vi "SPC_set_adjust_parameters.vi"(6 "SPC Adjust Parameters":T1={"vrt1"=64, "vrt2"=128, "vrt3"=192, "dith_g"=128, "gain_1"=1.0, "gain_2"=1.0, "gain_4"=1.0, "gain_8"=1.0, "tac_r0"=1.0, "tac_r1"=1.0, "tac_r2"=1.0, "tac_r4"=1.0, "tac_r8"=1.0, "sync_div"=0} {"sync_div" min=0 max=2; "tac_r8" format="%.2f"; "tac_r4" format="%.2f"; "tac_r2" format="%.2f"; "tac_r1" format="%.2f"; "tac_r0" format="%.2f"; "gain_8" format="%.2f"; "gain_4" format="%.2f"; "gain_2" format="%.2f"; "gain_1" format="%.2f"}, 8 "Error In":errorcluster, 10 "Module No":i16 min=0 max=7 step=1, 11 "DLL Path":path) -> (0 "Error Out":errorcluster, 2 "Module No":i16 min=0 max=7 step=1, 3 "DLL Path":path, 4 "actualSPC Adjust Parameters":T1={"vrt1"=64, "vrt2"=128, "vrt3"=192, "dith_g"=128, "gain_1"=1.0, "gain_2"=1.0, "gain_4"=1.0, "gain_8"=1.0, "tac_r0"=1.0, "tac_r1"=1.0, "tac_r2"=1.0, "tac_r4"=1.0, "tac_r8"=1.0, "sync_div"=0} {"sync_div" min=0 max=2; "tac_r8" format="%.2f"; "tac_r4" format="%.2f"; "tac_r2" format="%.2f"; "tac_r1" format="%.2f"; "tac_r0" format="%.2f"; "gain_8" format="%.2f"; "gain_4" format="%.2f"; "gain_2" format="%.2f"; "gain_1" format="%.2f"})   [LabVIEW 2019]
doc: "The adjust parameters in the internal DLL structures (not in the EEPROM) of the module ‘mod_no’ are set to values from the structure \"adjpara\". The function is used to set the module adjust parameters to values other than the values from the EEPROM. \nThe new adjust values will be used until the next call of SPC_init. The next call to SPC_init replaces the adjust parameters by the values from the EEPROM. We strongly discourage to use modified adjust parameters, because the module function can be seriously corrupted by wrong adjust values.\nThe structure \"SPC_Adjust_Para\" is defined in the file spcm_def.h.\n\ninfo@becker-hickl.com"
uses:
  SPC_Controls/SPC_adjust_para.ctl
panel:
  # "We strongly discourage to use modified adjust parameters, because the module function can be seriously corrupted by wrong adjust values."
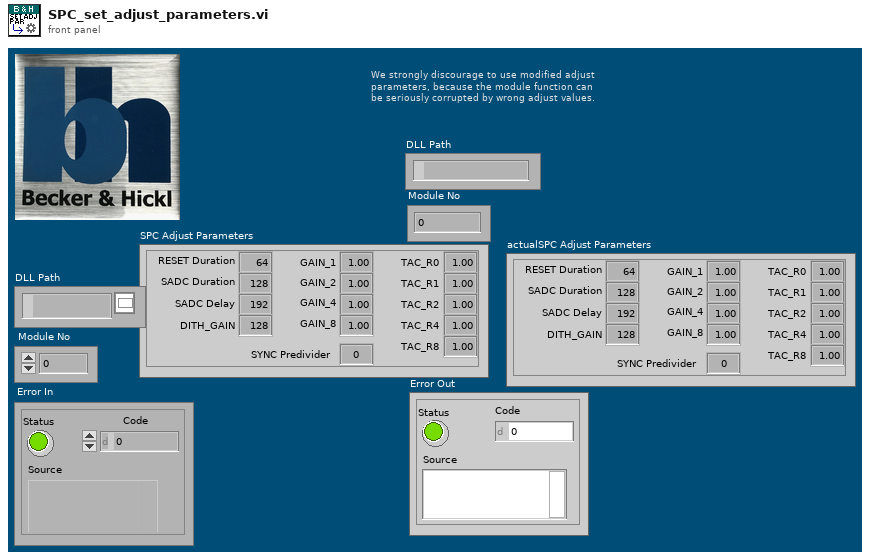
[diagram p1: front panel]
types:
  T1 = typedef "SPC_adjust_para.ctl" = cluster{"vrt1":i16, "vrt2":i16, "vrt3":i16, "dith_g":i16, "gain_1":sgl, "gain_2":sgl, "gain_4":sgl, "gain_8":sgl, "tac_r0":sgl, "tac_r1":sgl, "tac_r2":sgl, "tac_r4":sgl, "tac_r8":sgl, "sync_div":i16}
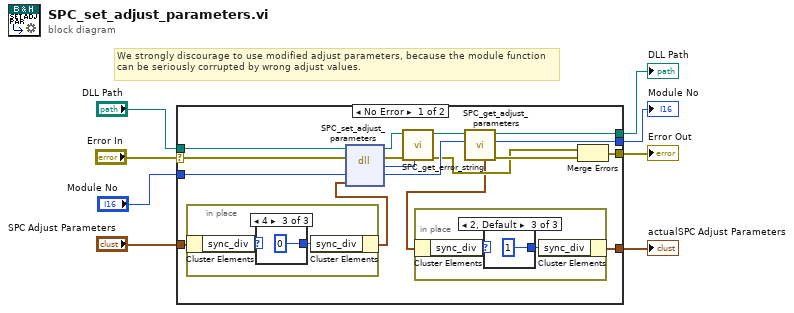
[diagram p0: block diagram]
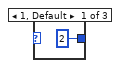
[diagram p2: hidden frame]
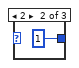
[diagram p3: hidden frame]
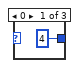
[diagram p4: hidden frame]
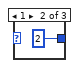
[diagram p5: hidden frame]
diagram:
  # "We strongly discourage to use modified adjust parameters, because the module function can be seriously corrupted by wrong adjust values."
  n1 = case shown="No Error" "Error In" {
    selector: "Error In" -> [w22 w38]
    tunnel: [w14 w38] -> w8
    tunnel: [w23 w39] -> w7
    tunnel: "DLL Path" -> [w21 w39]
    tunnel: "SPC Adjust Parameters" -> [w9 w37]
    tunnel: [w11 w37] -> w4
    tunnel: [w15 w36] -> w3
    tunnel: "Module No" -> [w17 w36]
    frame No Error {
      n2 = in-place {
        n3 = in-place-cluster #1(w9) -> ("sync_div"=w27:i16)
        n4 = case shown="4" w27 {
          tunnel: [i16 2 ("sync_div") i16 1 ("sync_div") i16 0 ("sync_div")] -> w26
          frame 1, Default {
          }
          frame 2 {
          }
          frame 4 {
          }
        }
        n5 = in-place-cluster #1("sync_div"=w26) -> (w10:T1)
      }
      n6 = dll-call lib="D:/spcm/lib/lab_view/lv10.0/spcm32.dll" fn="SPC_set_adjust_parameters"(path in=w21, error in=w22, "mod_no"=w17, w10) -> (path out=w19:path, error out=w25:errorcluster, "return type"=w20:i16, "mod_no"=w16:i16)  [unwired: 2 in]
      n7 = call "SPC_get_error_string.vi"("ErrorID"=w20, "Error In"=w25, "DLL Path"=w19) -> ("Error Out"=w13:errorcluster, "DLL Path"=w18:path)  [unwired: 6 in, 1 out]
      n8 = call "SPC_get_adjust_parameters.vi"("Module No"=w16, "DLL Path"=w18) -> ("Error Out"=w24:errorcluster, "Module No"=w15:i16, "DLL Path"=w23:path, "SPC adjust parameters"=w12:T1)  [unwired: 6 in]
      n9 = in-place {
        n10 = in-place-cluster #2(w12) -> ("sync_div"=w32:i16)
        n11 = case shown="2, Default" w32 {
          tunnel: [i16 4 ("sync_div") i16 2 ("sync_div") i16 1 ("sync_div")] -> w31
          frame 0 {
          }
          frame 1 {
          }
          frame 2, Default {
          }
        }
        n12 = in-place-cluster #2("sync_div"=w31) -> (w11:T1)
      }
      n13 = Merge Errors(w13, w24) -> (w14:errorcluster)
    }
    frame Error {
    }
  }
  "DLL Path" <- w7
  "Error Out" <- w8
  "actualSPC Adjust Parameters" <- w4
  "Module No" <- w3
